vi "GrabFrame.vi"(8 "error in (no error)":errorcluster, 10 "Image":u16[][](array[numeric]), 11 "InterferometryUI in":refnum<class "InterferometryUI.lvclass">) -> (0 "error out":errorcluster, 3 "InterferometryUI out":refnum<class "InterferometryUI.lvclass">)   [LabVIEW 2023, in "InterferometryUI.lvlib" / "InterferometryUI.lvclass"]
uses:
  InterferometryUI.lvclass
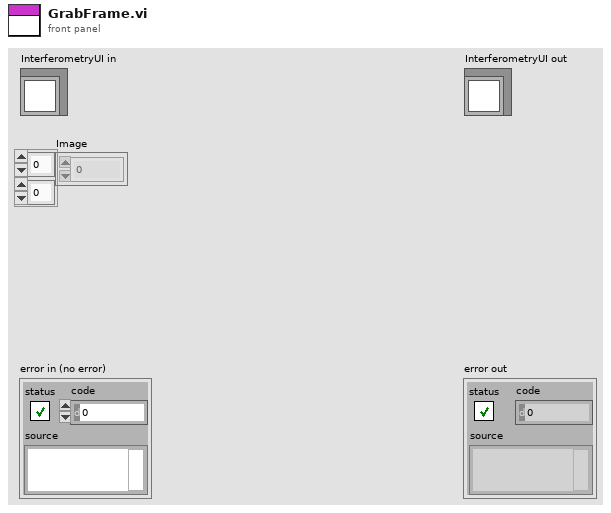
[diagram p1: front panel]
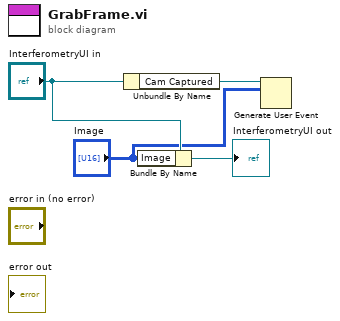
[diagram p0: block diagram]
diagram:
  n1 = Unbundle By Name("InterferometryUI in") -> ("Cam Captured"=w4:refnum<user-event>)
  n2 = Bundle By Name(cluster="InterferometryUI in", "Image"="Image") -> (→"InterferometryUI out":refnum<class "InterferometryUI.lvclass">)
  n3 = Generate User Event(user event=w4, event data cluster="Image") -> ()  [unwired: 2 in, 2 out]
